vi "ClassAppData.Load_Merge Data.vi"(7 "Merge(F)/Replace(T)":bool, 8 "error in (no error)":errorcluster, 10 "Data In":variant, 11 "Class - App Data in":refnum<class "Class.AppData.lvclass">) -> (0 "error out":errorcluster, 3 "Class - App Data out":refnum<class "Class.AppData.lvclass">)   [LabVIEW 2024, in "EQMF.lvlib" / "Config Utils.lvlib" / "Class.AppData.lvclass"]
doc: "<B>AppData Class:</B>\nThe AppData class keeps track of a library of data items that are used by an application. These data items have a name (text string) and value that can be any data type. \n\nThis VI takes in a variant with a list of data library items as attributes. It either merges the data with the existing data library or it replaces the data library in the class with the input data. \n<B>Merge(F)/Replace(T)</B> - This input is a Boolean that selects if the input data is to be merged or to be used to replace the existing data library."
uses:
  Class.AppData.lvclass
  Class.AppData.lvclass/Class.AppData.ctl
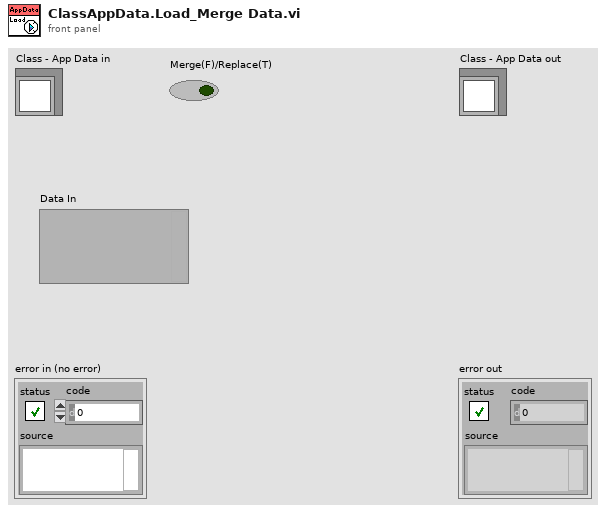
[diagram p1: front panel]
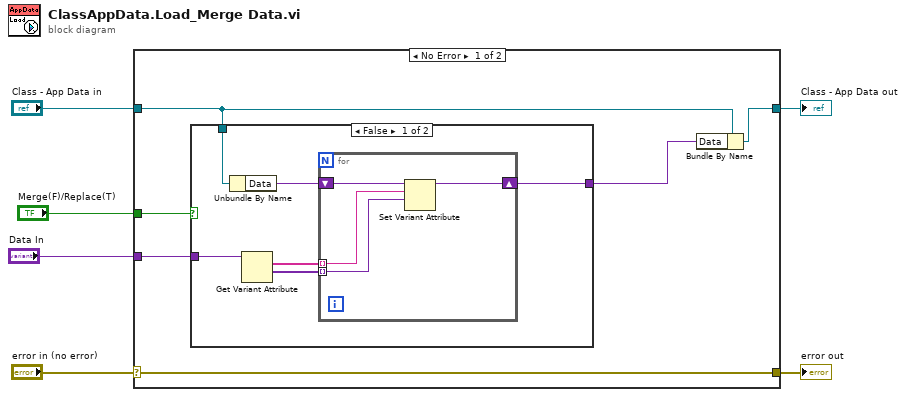
[diagram p0: block diagram]
diagram:
  n1 = case shown="No Error" "error in (no error)" {
    selector: "error in (no error)" -> [w7 w25]
    tunnel: [w7 w25] -> w5
    tunnel: [w12 w24] -> w3
    tunnel: "Class - App Data in" -> [w11 w24]
    tunnel: "Merge(F)/Replace(T)" -> [w10 _]
    tunnel: "Data In" -> [w8 _]
    frame No Error {
      n2 = case shown="False" w10 {
        tunnel: w11 -> [w18 _]
        tunnel: [w15 w23] -> w9
        tunnel: w8 -> [w17 w23]
        frame False {
          n3 = Unbundle By Name(w18) -> ("Data"=w16:variant)
          n4 = Get Variant Attribute(Variant=w17) -> (names=w14:string[], values=w13:variant[])  [unwired: 3 in, 2 out]
          n5 = for {
            shift-right: [w19] -> w15
            shift-left: w16 -> [w22]
            tunnel: w14 -> [w21] mode=indexing
            tunnel: w13 -> [w20] mode=indexing
            n6 = Set Variant Attribute(Variant=w22, name=w21, value=w20) -> (Variant out=w19:variant)  [unwired: 1 in, 2 out]
          }
        }
        frame True {
        }
      }
      n7 = Bundle By Name(cluster=w11, "Data"=w9) -> (w12:refnum<class "Class.AppData.lvclass">)
    }
    frame Error {
    }
  }
  "error out" <- w5
  "Class - App Data out" <- w3
